vi "Parse.vi"(8 "error in":errorcluster, 11 "Lv Proj Document Type:TAF Proj":refnum<class "TAF Proj.lvclass">) -> (0 "error out":errorcluster, 3 "Lv Proj Document Type:TAF Proj":refnum<class "TAF Proj.lvclass">)   [LabVIEW 2021, in "TAF Proj Document Type.lvlib" / "TAF Proj.lvclass"]
uses:
  <vilib>/Wovalab/AntiDoc/Document Type/Add-ons/LabVIEW TAF Project/TAF Proj/TAF Proj.lvclass
  C:/Program Files (x86)/National Instruments/LabVIEW 2021/vi.lib/Wovalab/AntiDoc/Document Type/Document/Document Type.lvclass
  <vilib>/Wovalab/AntiDoc/Document Type/Add-ons/LabVIEW TAF Project/TAF Proj Config/TAF Proj Config.lvclass
  <vilib>/Wovalab/AntiDoc/Document Type/Add-ons/LabVIEW TAF Project/TAF Proj/TAF Proj.lvclass/TAF Proj.ctl
  <vilib>/Wovalab/AntiDoc/Document Type/Document/Document Type.lvclass/Document Type.ctl
  <vilib>/Wovalab/AntiDoc/Document Type/Document/Read Config.vi
  <vilib>/Wovalab/AntiDoc/Document Type/Config/Config.lvclass
  <vilib>/Wovalab/AntiDoc/Document Type/Add-ons/LabVIEW TAF Project/Project Parser/Project Parser.lvlib
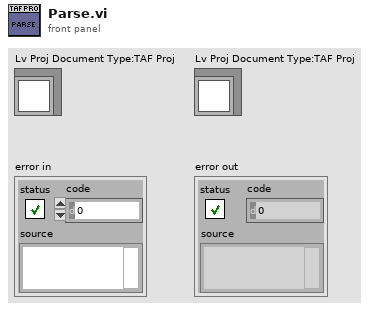
[diagram p1: front panel]
types:
  T1 = typedef "TAF Proj Document Type.lvlib/Project Parser.lvlib/Target--cluster.ctl" = cluster{"Name":string, "Blocs":T2}
  T2 = typedef "TAF Proj Document Type.lvlib/Project Parser.lvlib/Blocs--cluster.ctl" = cluster{"DQMH Modules":refnum<class "Dqmh Module.lvclass">[], "LVClasses":refnum<class "Class.lvclass">[], "Other Libraries":refnum<class "Lib.lvclass">[], "Custom Errors":refnum<class "Custom Errors.lvclass">, "Classes Overview":refnum<class "Classes Overview.lvclass">, "Dqmh Modules Overview":refnum<class "Dqmh Modules Overview.lvclass">, "TAFIFConfiguration":refnum<class "TAFConfiguration.lvclass">[], "FrontPanelGUIOut":refnum<class "FrontPanelGUI.lvclass">}
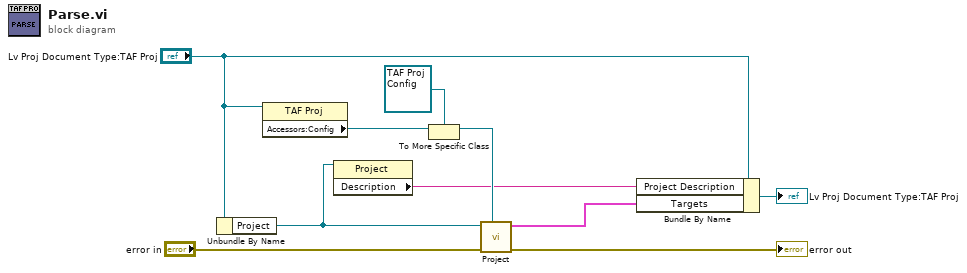
[diagram p0: block diagram]
diagram:
  n1 = Unbundle By Name("Lv Proj Document Type:TAF Proj") -> ("Project"=w2:refnum<vi>)
  n2 = property class="TAF Proj"(reference="Lv Proj Document Type:TAF Proj") -> ("Accessors:Config"=w5:refnum<class "Config.lvclass">)  [unwired: 1 in, 2 out]
  n3 = property class="Project"(reference=w2) -> ("Description"=w1:string)  [unwired: 1 in, 2 out]
  n4 = To More Specific Class(target class=refnum<class "TAF Proj Config.lvclass"> refnum ("Lv Proj Document Type.lvlib:Config"), reference=w5) -> (specific class reference=w4:refnum<class "TAF Proj Config.lvclass">)  [unwired: 1 in, 1 out]
  n5 = call <vilib>:"Project.vi"("Config in"=w4, "error in"="error in", "Project"=w2) -> ("error out"=→"error out":errorcluster, "Targets"=w7:T1[])  [unwired: 7 in]
  n6 = Bundle By Name(cluster="Lv Proj Document Type:TAF Proj", "Project Description"=w1, "Targets"=w7) -> (→"Lv Proj Document Type:TAF Proj":refnum<class "TAF Proj.lvclass">)
